vi "Settings_TestCase_TestCaseDuplicate.vi"(8 "error in":errorcluster, 11 "VI Server Cluster":T1) -> (0 "error out":errorcluster, 2 "Update?":bool, 3 "VI Server ClusterDUP":T1)   [LabVIEW 2020]
uses:
  Instruments/NA-E5071B/E5071B.llb/Recover Text Ring U16.vi
  Instruments/NA-E5071B/E5071B.llb/Labels&Control References.ctl
panel:
  in  "SourceTestCase":u16(ring) caption="Copy Test Case" items=["1.1", "1.2", "1.3", "1.4"]
  in  "Duplicate":bool
  in  "Cancel":bool
  in  "TestCase":u16(ring) caption="To Test Case" items=["1.1", "1.2", "1.3", "1.4"]
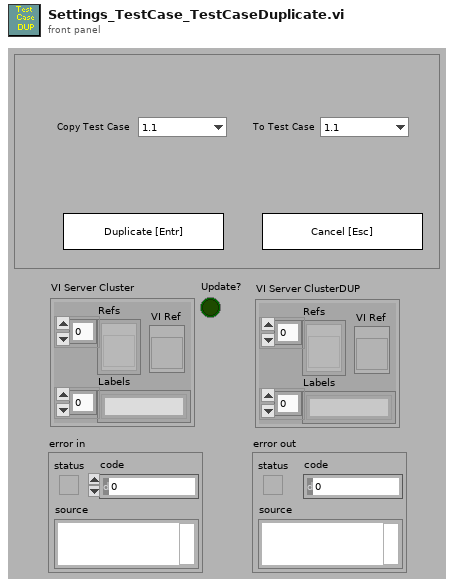
[diagram p1: front panel]
types:
  T1 = typedef "Labels&Control References.ctl" = cluster{"Refs":refnum<vi>[], "Labels":string[], "VI Ref":refnum<vi>}
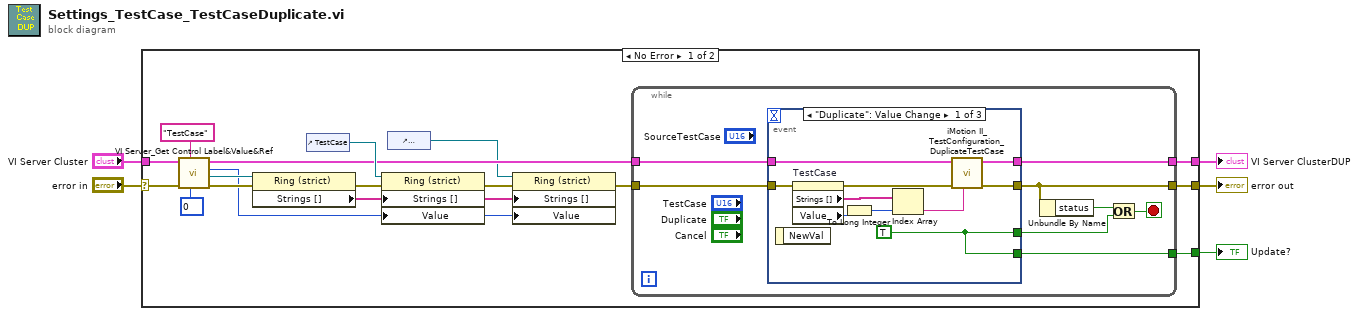
[diagram p0: block diagram]
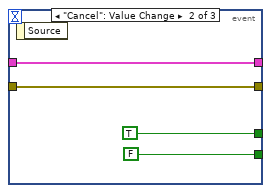
[diagram p2: hidden frame]
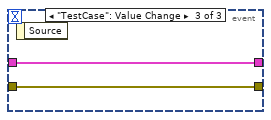
[diagram p3: hidden frame]
diagram:
  n1 = case shown="No Error" "error in" {
    selector: "error in" -> [w17 w47]
    tunnel: [w22 w47] -> w5
    tunnel: "VI Server Cluster" -> [w15 _]
    tunnel: [w19 _] -> w2
    tunnel: [w18 _] -> w1
    frame No Error {
      w11 = u16 0 items=["", "1", "2", "3", "4", "5", "6", "7", "8", "9", "10", "11", "12", "13", "14", "15", "16", "17", "18", "19", "20", "21", "22", "23", "24", "25", "26", "27", "28", "29", "30", "31", "32", "33", "34", "35", "36", "37", "38", "39", "40", "41", "42", "43", "44", "45", "46", "47", "48", "49", "50", "51", "52", "53", "54", "55", "56", "57", "58", "59", "60", "61", "62", "63", "64", "65", "66", "67", "68", "69", "70", "71", "72", "73", "74", "75", "76", "77", "78", "79", "80", "81", "82", "83", "84", "85", "86", "87", "88", "89", "90", "91", "92", "93", "94", "95", "96", "97", "98", "99", "100", "101", "102", "103", "104", "105", "106", "107", "108", "109", "110", "111", "112", "113", "114", "115", "116", "117", "118", "119", "120", "121", "122", "123", "124", "125", "126", "127", "128", "129", "130", "131", "132", "133", "134", "135", "136", "137", "138", "139", "140", "141", "142", "143", "144", "145", "146", "147", "148", "149", "150", "151", "152", "153", "154", "155", "156", "157", "158", "159", "160", "161", "162", "163", "164", "165", "166", "167", "168", "169", "170"] ("SourceTestCase")
      n2 = call-poly "VI Server_Get Control Label&Value&Ref.vi"("Default Value"=w11, "Label"="TestCase", "error in"=w17, "Data Cluster"=w15) -> ("error out"=w16:errorcluster, "Control Ref"=w14:refnum<vi>, "Value"=w7:u16, "Data Cluster dup"=w13:T1)  [unwired: 3 in, 1 out]
      n3 = property class="Ring (strict)"(reference=w14, error in=w16) -> (error out=w21:errorcluster, "Strings []"=w8:string[])  [unwired: 1 out]
      n4 = control-ref of="TestCase"() -> (w20:refnum<vi>)
      n5 = property class="Ring (strict)"(reference=w20, error in=w21, "Strings []"=w8, "Value"=w7) -> (error out=w10:errorcluster)  [unwired: 1 out]
      n6 = control-ref of="SourceTestCase"() -> (w6:refnum<vi>)
      n7 = property class="Ring (strict)"(reference=w6, error in=w10, "Strings []"=w8, "Value"=w7) -> (error out=w9:errorcluster)  [unwired: 1 out]
      n8 = while {
        tunnel: [w28] -> w22
        tunnel: w9 -> [w30]
        tunnel: w13 -> [w29]
        tunnel: [w24] -> w19
        tunnel: [w23] -> w18
        stop <- w26 stop-if-true
        n9 = event shown="[0] \"Duplicate\": Value Change" {
          selector: _ -> [_ _ _]
          dyn-events: _ -> [_ _ _]
          timeout: _ -> [_ _ _]
          tunnel: [w40 w44 w46] -> w28
          tunnel: w30 -> [w38 w44 w46]
          tunnel: w29 -> [w39 w42 w45]
          tunnel: [w31 TRUE _] -> w25
          tunnel: [w32 w42 w45] -> w24
          tunnel: [w31 FALSE _] -> w23
          event "Duplicate": Value Change {
            w31 = TRUE
            n10 = event-data() -> ()  [unwired: 1 in, 1 out]
            n11 = property on="TestCase" class="Ring (strict)"(error in=w38) -> (error out=w37:errorcluster, "Strings []"=w36:string[], "Value"=w35:u16)  [unwired: 1 in, 1 out]
            n12 = To Long Integer(number=w35) -> (32bit integer=w33:i32)
            n13 = Index Array(array=w36, index=w33) -> (element=w34:string)
            n14 = call "iMotion II_TestConfiguration_DuplicateTestCase.vi"("Selection"=w34, "error in (no error)"=w37, "Data Cluster"=w39) -> ("error out"=w40:errorcluster, "Data Cluster DUP"=w32:T1)  [unwired: 7 in]
          }
          event "Cancel": Value Change {
            n15 = event-data() -> ()  [unwired: 1 in, 1 out]
          }
          event "TestCase": Value Change {
            n16 = event-data() -> ()  [unwired: 1 in, 1 out]
          }
        }
        n17 = Unbundle By Name(w28) -> ("status"=w27:bool)
        n18 = Or(x=w27, y=w25) -> (x .or. y?=w26:bool)
      }
    }
    frame Error {
    }
  }
  "error out" <- w5
  "VI Server ClusterDUP" <- w2
  "Update?" <- w1
